vi "Analogue 2 Direct.vi"(1 "att 7":fxp<+/-,20,5>, 2 "att 6":fxp<+/-,20,5>, 3 "att 5":fxp<+/-,20,5>, 8 "att 4":fxp<+/-,20,5>, 9 "att 3":fxp<+/-,20,5>, 10 "att 2":fxp<+/-,20,5>, 11 "att 1":fxp<+/-,20,5>) -> ()   [LabVIEW 2023]
uses:
  <vilib>/rvi/eio/common/nirviEmuTemplateMethod_errors.vi
  <vilib>/eio/EIONode/EIONode.xnode
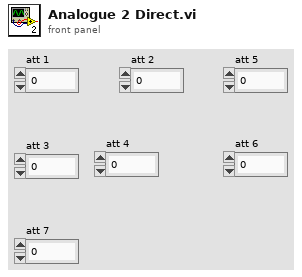
[diagram p1: front panel]
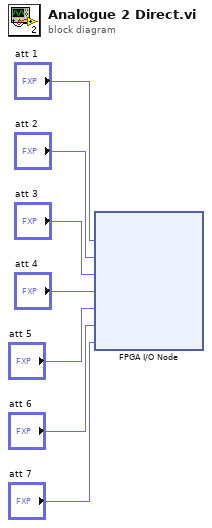
[diagram p0: block diagram]
diagram:
  n1 = xnode "FPGA I/O Node"("Mod3/AO6"="att 1", "Mod3/AO7"="att 2", "Mod3/AO8"="att 3", "Mod3/AO9"="att 4", "Mod3/AO10"="att 5", "Mod3/AO11"="att 6", "Mod3/AO12"="att 7") -> ()  [unwired: 7 in, 7 out]
